vi "Charger_Open.vi"(4 "error in":errorcluster, 6 "delay after config (100 ms)":dbl[unit]=0.1 format="%_3p", 7 "Charger COM port":refnum<visa-resource-name>="COM7") -> (0 "error out":errorcluster)   [LabVIEW 2020]
doc: "This function configures the Charger Test Set serial port with no termination character and the normal serial port default parameters, then waits for 100 ms."
uses:
  <vilib>/Instr/_visa.llb/VISA Configure Serial Port (Instr).vi
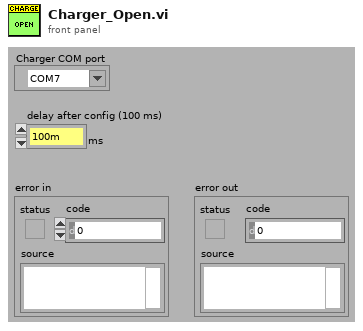
[diagram p1: front panel]
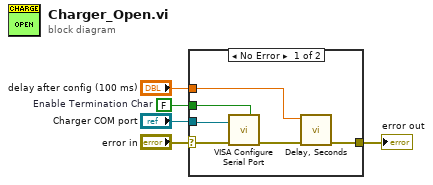
[diagram p0: block diagram]
diagram:
  w4 = FALSE  # Enable Termination Char
  n1 = case shown="No Error" "error in" {
    selector: "error in" -> [w9 w12]
    tunnel: [w11 w12] -> w5
    tunnel: w4 -> [w10 _]
    tunnel: "Charger COM port" -> [w7 _]
    tunnel: "delay after config (100 ms)" -> [w6 _]
    frame No Error {
      n2 = call-poly "VISA Configure Serial Port"("VISA resource name"=w7, "Enable Termination\nChar (T)"=w10, "error in (no error)"=w9) -> ("error out"=w8:errorcluster)  [unwired: 11 in, 1 out]
      n3 = call "Delay, Seconds.vi"("error in"=w8, "delay"=w6) -> ("error out"=w11:errorcluster)  [unwired: 5 in, 1 out]
    }
    frame Error {
    }
  }
  "error out" <- w5
